vi "二进制文件（读取二进制文件函数）.vi"() -> ()   [LabVIEW 2017]
panel:
  out "波形图":dbl[](graph)
  out "写入数组长度":i32[](array[numeric])
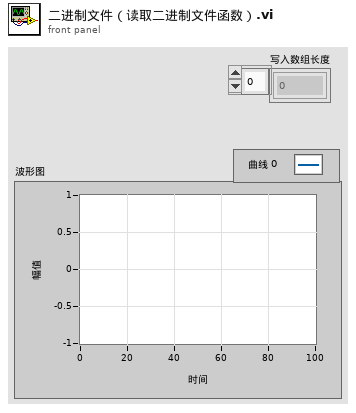
[diagram p1: front panel]
types:
  T1 = enum16{"open", "replace", "create", "open or create", "replace or create", "replace or create with confirmation"}
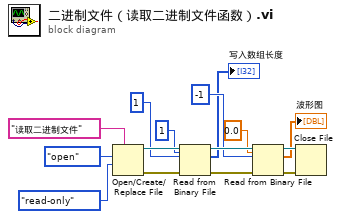
[diagram p0: block diagram]
diagram:
  n1 = Open/Create/Replace File(prompt="读取二进制文件" ("提示"), operation (0:open)=T1."open" ("操作(0:open)"), access (0:read/write)=enum16{"read/write", "read-only", "write-only"}."read-only" ("权限(0:read/write)")) -> (refnum out=w12:refnum<file>, error out=w11:errorcluster)  [unwired: 3 in, 1 out]
  n2 = Read from Binary File(5:1 ("总数(1)"), 8:w11, 10:1 ("总数(1)"), 11:w12) -> (0:w8:errorcluster, 2:→"写入数组长度":i32[], 3:w9:refnum<file>)  [unwired: 2 in, 1 out]
  n3 = Read from Binary File(5:0.0, 8:w8, 10:-1 ("总数(1)"), 11:w9) -> (0:w6:errorcluster, 2:→"波形图":dbl[], 3:w7:refnum<file>)  [unwired: 2 in, 1 out]
  n4 = Close File(refnum=w7, error in=w6) -> ()  [unwired: 2 out]
